vi "SendTCPPort.vi"(8 "error in (no error)":errorcluster, 11 "TCP Com in":refnum<class "TCP Com.lvclass">) -> (0 "error out":errorcluster, 3 "TCP Com out":refnum<class "TCP Com.lvclass">)   [LabVIEW 2023, in "TCP Com.lvclass"]
uses:
  TCP Com.lvclass
  C:/Users/santharu.subramanian/Desktop/LOA New/Documents/LV New Assignments/Sender-Receiver/Classes/Communication/Communication.lvclass
  Data/Data.lvclass
  TCP Com.lvclass/TCP Com.ctl
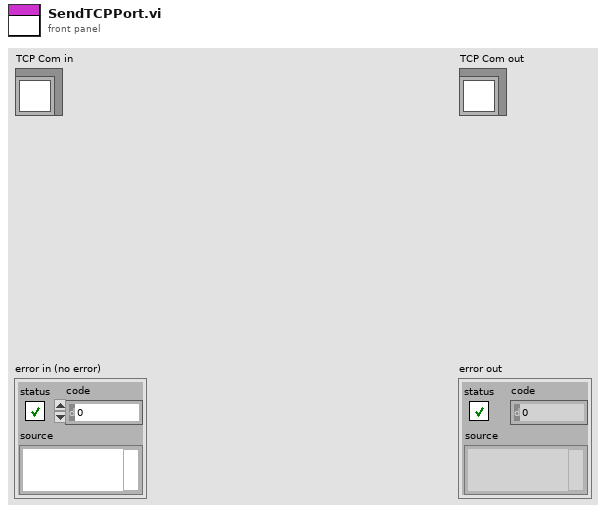
[diagram p1: front panel]
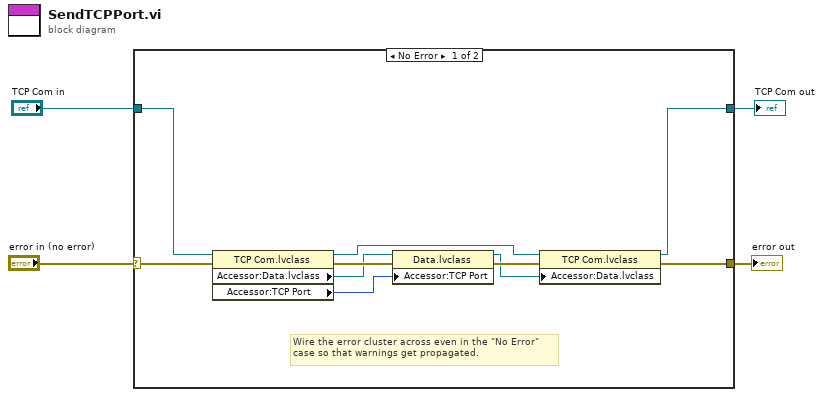
[diagram p0: block diagram]
diagram:
  n1 = case shown="No Error" "error in (no error)" {
    selector: "error in (no error)" -> [w14 w16]
    tunnel: [w5 w16] -> w3
    tunnel: [w6 w15] -> w1
    tunnel: "TCP Com in" -> [w12 w15]
    frame No Error {
      # "Wire the error cluster across even in the \"No Error\"\ncase so that warnings get propagated."
      n2 = property class="TCP Com.lvclass"(reference=w12, error in=w14) -> (reference out=w8:refnum<class "TCP Com.lvclass">, error out=w13:errorcluster, "Accessor:Data.lvclass"=w11:refnum<class "Data.lvclass">, "Accessor:TCP Port"=w10:u16)
      n3 = property class="Data.lvclass"(reference=w11, error in=w13, "Accessor:TCP Port"=w10) -> (reference out=w7:refnum<class "Data.lvclass">, error out=w9:errorcluster)
      n4 = property class="TCP Com.lvclass"(reference=w8, error in=w9, "Accessor:Data.lvclass"=w7) -> (reference out=w6:refnum<class "TCP Com.lvclass">, error out=w5:errorcluster)
    }
    frame Error {
    }
  }
  "error out" <- w3
  "TCP Com out" <- w1
